vi "Agilent DMM Read Trigger Source.vi"(8 "error in (no error)":errorcluster, 11 "VISA Resource Name":refnum<visa-resource-name>) -> (0 "error out":errorcluster, 2 "Trigger Source":T1, 3 "dup VISA Resource Name":refnum<visa-resource-name>)   [LabVIEW 2011]
doc: "This VI for the HP 8753 is used to read the sweep type.\n\n0 LINEAR FREQ\n1 LOG FREQ\n2 LIST FREQ\n3 CW TIME\n4 POWER SWEEP"
uses:
  TypeDefs/Agilent DMM Trigger Source.ctl
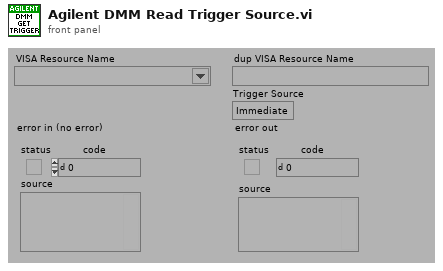
[diagram p1: front panel]
types:
  T1 = typedef "Agilent DMM Trigger Source.ctl" = enum16{"Immediate", "Bus", "External"}
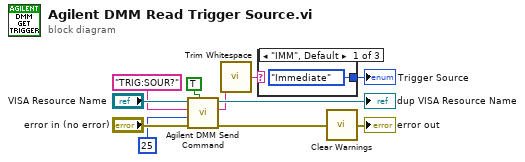
[diagram p0: block diagram]
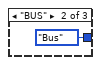
[diagram p2: hidden frame]
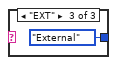
[diagram p3: hidden frame]
diagram:
  n1 = call "Agilent DMM Send Command.vi"("Read? (F)"=TRUE, "error in (no error)"="error in (no error)", "Byte Count"=u32 25 ("byte count"), "Command"="TRIG:SOUR?" ("write buffer"), "VISA Resource Name"="VISA Resource Name") -> ("error out"=w4:errorcluster, "Data Read"=w3:string, "dup VISA Resource Name"=→"dup VISA Resource Name":refnum<visa-resource-name>)  [unwired: 4 out]
  n2 = call <vilib>:"Trim Whitespace.vi"("string"=w3) -> ("trimmed string"=w7:string)  [unwired: 1 in]
  n3 = case shown="\"IMM\", Default" w7 {
    tunnel: [Agilent_DMM_Trigger_Source."Immediate" ("Trigger Source") Agilent_DMM_Trigger_Source."Bus" ("Trigger Source") Agilent_DMM_Trigger_Source."External" ("Trigger Source")] -> w8
    frame "IMM", Default {
    }
    frame "BUS" {
    }
    frame "EXT" {
    }
  }
  "Trigger Source" <- w8
  n4 = call "Clear Warnings.vi"("error in (no error)"=w4) -> ("error out"=→"error out":errorcluster)
